vi "ImagesEnumsToPictures.vi"(8 "error in (no error)":errorcluster, 11 "BoardDisplay in":refnum<class "BoardDisplay.lvclass">) -> (0 "error out":errorcluster, 3 "BoardDisplay out":refnum<class "BoardDisplay.lvclass">)   [LabVIEW 2015, in "TronviewPresentation.lvlib" / "BoardDisplay.lvclass"]
uses:
  BoardDisplay.lvclass
  TronviewGame/GameRecorder/GameRecorder.lvclass
  TronviewGame/Board/Board.lvclass
panel:
  out "Array 3":picture[][](array[picture])=[[bytes[1905], bytes[1905], bytes[1905], bytes[1905], bytes[1905], bytes[1905], bytes[1905], bytes[1905], bytes[1905], bytes[1905], bytes[1905], bytes[1905], bytes[1905], bytes[1905], bytes[1905], bytes[1905]], [bytes[1905], bytes[1905], bytes[1905], bytes[1905], bytes[1905], bytes[1905], bytes[1905], bytes[1905], bytes[1905], bytes[1905], bytes[1905], bytes[1905], bytes[1905], bytes[1905], bytes[1905], bytes[1905]], [bytes[1905], bytes[1905], bytes[2005], bytes[1905], bytes[1905], bytes[1905], bytes[1905], bytes[1905], bytes[1905], bytes[1905], bytes[1905], bytes[1905], bytes[1905], bytes[1905], bytes[1905], bytes[1905]], [bytes[1905], bytes[1905], bytes[2005], bytes[1905], bytes[1905], bytes[1905], bytes[1905], bytes[1905], bytes[1905], bytes[1905], bytes[1905], bytes[1905], bytes[1905], bytes[1905], bytes[1905], bytes[1905]], [bytes[1905], bytes[1905], bytes[2005], bytes[1905], bytes[1905], bytes[1905], bytes[1905], bytes[1905], bytes[1905], bytes[1905], bytes[1905], bytes[1905], bytes[1905], bytes[1905], bytes[1905], bytes[1905]], [bytes[1905], bytes[1905], bytes[2005], bytes[2005], bytes[1905], bytes[1905], bytes[1905], bytes[1905], bytes[1905], bytes[1905], bytes[1905], bytes[1905], bytes[1905], bytes[1905], bytes[1905], bytes[1905]], [bytes[2005], bytes[2005], bytes[2005], bytes[2005], bytes[1905], bytes[1905], bytes[1905], bytes[1905], bytes[1905], bytes[1905], bytes[1905], bytes[1905], bytes[1905], bytes[1905], bytes[1905], bytes[1905]], [bytes[2005], bytes[2005], bytes[2005], bytes[1905], bytes[1905], bytes[1905], bytes[1905], bytes[1905], bytes[1905], bytes[1905], bytes[1905], bytes[1905], bytes[1905], bytes[1905], bytes[1905], bytes[1905]], [bytes[2005], bytes[2005], bytes[2005], bytes[1905], bytes[2005], bytes[2005], bytes[1905], bytes[1905], bytes[1905], bytes[1905], bytes[1905], bytes[1905], bytes[1905], bytes[1905], bytes[1905], bytes[1905]], [bytes[1905], bytes[1905], bytes[2005], bytes[2005], bytes[2005], bytes[2005], bytes[2005], bytes[1905], bytes[1905], bytes[1905], bytes[1905], bytes[1905], bytes[1905], bytes[1905], bytes[1905], bytes[1905]], [bytes[1905], bytes[1905], bytes[2005], bytes[2005], bytes[1905], bytes[1905], bytes[2005], bytes[1905], bytes[1905], bytes[1905], bytes[1905], bytes[1905], bytes[1905], bytes[1905], bytes[1905], bytes[1905]], [bytes[2005], bytes[2005], bytes[2005], bytes[2005], bytes[2005], bytes[2005], bytes[2005], bytes[1905], bytes[1905], bytes[1905], bytes[1905], bytes[1905], bytes[1905], bytes[1905], bytes[1905], bytes[1905]], [bytes[2005], bytes[2005], bytes[2005], bytes[2005], bytes[2005], bytes[2005], bytes[2005], bytes[2005], bytes[2005], bytes[1905], bytes[1905], bytes[1905], bytes[1905], bytes[1905], bytes[1905], bytes[1905]], [bytes[2005], bytes[2005], bytes[1905], bytes[1905], bytes[2005], bytes[2005], bytes[2005], bytes[2005], bytes[2005], bytes[1905], bytes[1905], bytes[1905], bytes[1905], bytes[1905], bytes[1905], bytes[1905]], [bytes[1905], bytes[1905], bytes[1905], bytes[1905], bytes[1905], bytes[1905], bytes[1905], bytes[1905], bytes[1905], bytes[1905], bytes[1905], bytes[1905], bytes[1905], bytes[1905], bytes[1905], bytes[1905]], [bytes[1905], bytes[1905], bytes[1905], bytes[1905], bytes[1905], bytes[1905], bytes[1905], bytes[1905], bytes[1905], bytes[1905], bytes[1905], bytes[1905], bytes[1905], bytes[1905], bytes[1905], bytes[1905]]]
  out "Array 2":picture[][](array[picture])
  in  "ImagesFolder":path
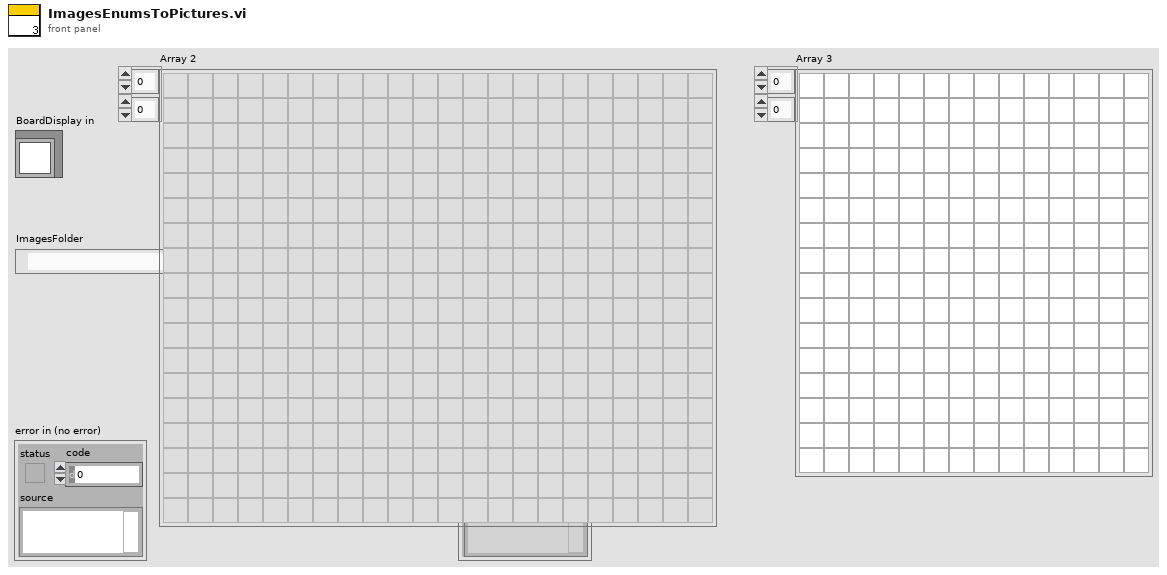
[diagram p1: front panel]
types:
  T1 = typedef "TronviewGame.lvlib/Board.lvclass/Position.ctl" = cluster{"Column":i32, "Row":i32}
  T2 = typedef "TronviewPresentation.lvlib/BoardDisplay.lvclass/TrajectoryField.ctl" = enum16{"Empty", "NS", "NE", "NW", "EW", "SE", "SW"}
  T3 = typedef "TronVIEWBotAPI.lvlib/MovementDirection.ctl" = enum16{"N", "S", "W", "E"}
  T4 = typedef "imagedata.ctl" = cluster{"image type":i32, "image depth":i32, "image":u8[], "mask":u8[], "colors":u32[], "Rectangle":cluster{"left":i16, "top":i16, "right":i16, "bottom":i16}}
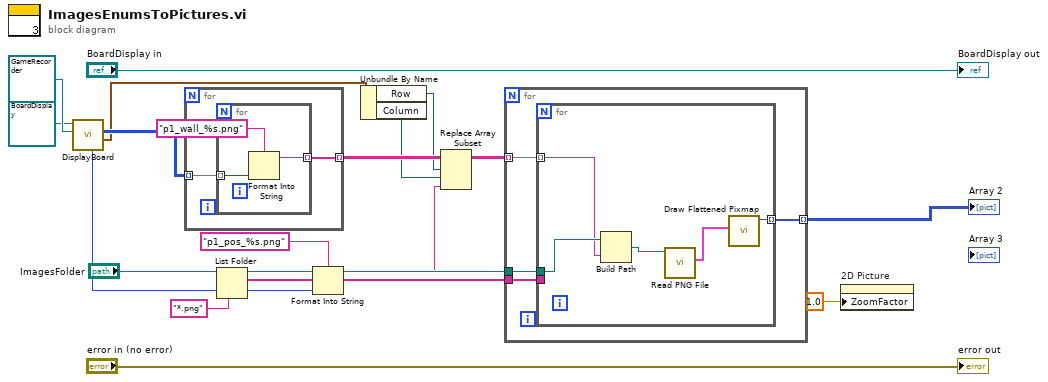
[diagram p0: block diagram]
diagram:
  n1 = call "DisplayBoard.vi"("GameRecorder"=refnum<class "GameRecorder.lvclass"> refnum, "BoardDisplay in"=refnum<class "BoardDisplay.lvclass"> refnum) -> ("PlayerFinalPosition"=w6:T1, "Array"=w8:T2[][], "PlayerFinalDirection"=w3:T3)  [unwired: 5 in, 2 out]
  n2 = for {
    tunnel: w8 -> [w21] mode=indexing
    tunnel: [w20] -> w13 mode=indexing
    n3 = for {
      tunnel: w21 -> [w24] mode=indexing
      tunnel: [w22] -> w20 mode=indexing
      n4 = Format Into String(format string="p1_wall_%s.png", w24) -> (resulting string=w22:string)  [unwired: 2 in, 1 out]
    }
  }
  n5 = List Folder(path="ImagesFolder", pattern="*.png") -> (path out=w14:path, filenames=w15:string[])  [unwired: 2 in, 2 out]
  n6 = Format Into String(format string="p1_pos_%s.png", w3) -> (resulting string=w2:string)  [unwired: 2 in, 1 out]
  n7 = Unbundle By Name(w6) -> ("Row"=w5:i32, "Column"=w4:i32)
  n8 = Replace Array Subset(array=w13, new element=w2, index (row)=w5, index (col)=w4) -> (w7:string[][])
  n9 = for {
    tunnel: w15 -> [w26]
    tunnel: w14 -> [w27]
    tunnel: w7 -> [w28] mode=indexing
    tunnel: [w25] -> w12 mode=indexing
    n10 = for {
      tunnel: w28 -> [w32] mode=indexing
      tunnel: w27 -> [w33]
      tunnel: w26 -> [_]
      tunnel: [w29] -> w25 mode=indexing
      n11 = Build Path(base path=w33, name or relative path=w32) -> (appended path=w31:path)
      n12 = call <vilib>:"Read PNG File.vi"("path to PNG file"=w31) -> ("image data"=w30:T4)  [unwired: 8 in, 2 out]
      n13 = call <vilib>:"Draw Flattened Pixmap.vi"("image data"=w30) -> ("new picture"=w29:picture)  [unwired: 8 in]
    }
  }
  "Array 2" <- w12
  n14 = property on="2D Picture" class="Pict"("ZoomFactor"=sgl 1.0 ("Zoom Factor")) -> ()  [unwired: 2 in, 2 out]
  "error out" <- "error in (no error)"
  "BoardDisplay out" <- "BoardDisplay in"
